vi "Pre Launch Init.vi"(11 "Cylinder in":refnum<class "Cylinder.lvclass">) -> (0 "error out":errorcluster, 3 "Cylinder out":refnum<class "Cylinder.lvclass">)   [LabVIEW 2015, in "cRIO-Carbondioxide.lvlib" / "CO2-Actor.lvlib" / "Cylinder.lvclass"]
doc: "(<B>Filename</B>: Actor Framework.lvlib:Actor.lvclass:Pre Launch Init.vi)\n\nDefines behavior that occurs after the Launch Actor method is invoked but before the actor's Actor Core method begins running.\n\nThe Pre Launch Init method is guaranteed to finish before the Launch Actor method returns to its caller and before the actor itself receives any messages. Any references that the Pre Launch Init method obtains are guaranteed to have the same lifetime as the actor itself. Any errors that the Pre Launch Init method returns will abort the launch.\n\nBy default, this method does nothing. A descendant class may override it to define behavior."
uses:
  Cylinder.lvclass
  Cylinder.lvclass/Cylinder.ctl
  <vilib>/ActorFramework/Actor/Actor.lvclass/Actor.ctl
  <vilib>/ActorFramework/Message Enqueuer/Message Enqueuer.lvclass/Message Enqueuer.ctl
  Cylinder Messages/Home Msg/Home Msg.lvclass/Home Msg.ctl
  <vilib>/ActorFramework/Actor/Read Self Enqueuer.vi
  <vilib>/ActorFramework/Message Enqueuer/Enqueue.vi
  <vilib>/ActorFramework/Message Enqueuer/Init from Existing Queue.vi
  <vilib>/ActorFramework/Message Priority Queue/Priority Enqueue.vi
  CO2 Actor/CO2 Actor.lvclass
  Cylinder Messages/Home Msg/Home Msg.lvclass
  Interlocks/Interlock Chain/Interlock Chain.lvclass
  CO2 Actor Messages/Launch Nested Actors Msg/Launch Nested Actors Msg.lvclass
  <vilib>/ActorFramework/Message Enqueuer/Message Enqueuer.lvclass
  <vilib>/ActorFramework/Actor/Actor.lvclass
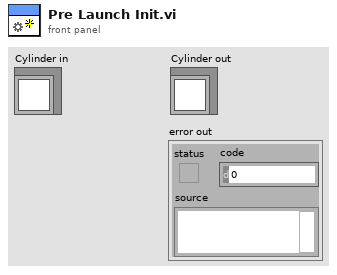
[diagram p1: front panel]
types:
  T1 = cluster{"Read Access":enum8{"Allowed", "Required", "None"}, "Write Access":enum8{"Allowed", "Required", "None"}}
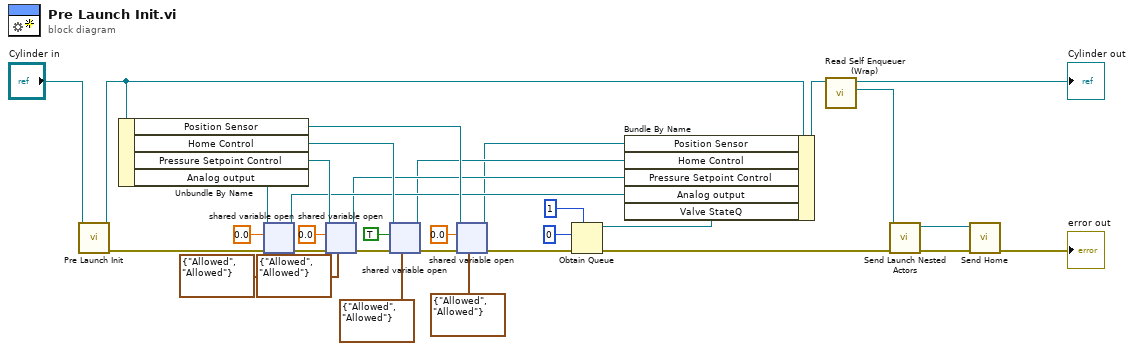
[diagram p0: block diagram]
diagram:
  n1 = call-parent "Pre Launch Init.vi"("CO2 Actor in"="Cylinder in") -> ("error out"=w30:errorcluster, "CO2 Actor out"=w26:refnum<class "Cylinder.lvclass">)  [unwired: 9 in]
  n2 = Unbundle By Name(w26) -> ("Position Sensor"=w9:refnum<k21>, "Home Control"=w16:refnum<k21>, "Pressure Setpoint Control"=w27:refnum<k21>, "Analog output"=w29:refnum<k21>)
  n3 = shared-variable-open(w29, w30, 0.0 ("data type"), T1 {"Read Access"=enum."Allowed", "Write Access"=enum."Allowed"} ("access")) -> (w5:refnum<k21>, w28:errorcluster)
  n4 = shared-variable-open(w27, w28, 0.0, T1 {"Read Access"=enum."Allowed", "Write Access"=enum."Allowed"} ("access")) -> (w4:refnum<k21>, w17:errorcluster)
  n5 = shared-variable-open(w16, w17, TRUE, T1 {"Read Access"=enum."Allowed", "Write Access"=enum."Allowed"} ("access")) -> (w3:refnum<k21>, w10:errorcluster)
  n6 = shared-variable-open(w9, w10, 0.0 ("data type"), T1 {"Read Access"=enum."Allowed", "Write Access"=enum."Allowed"} ("access")) -> (w2:refnum<k21>, w6:errorcluster)
  n7 = Obtain Queue(max queue size (-1, unlimited)=1, element data type=u16 0 ("element"), error in (no error)=w6) -> (queue out=w1:refnum<queue>, error out=w19:errorcluster)  [unwired: 2 in, 1 out]
  n8 = Bundle By Name(cluster=w26, "Position Sensor"=w2, "Home Control"=w3, "Pressure Setpoint Control"=w4, "Analog output"=w5, "Valve StateQ"=w1) -> (w21:refnum<class "Cylinder.lvclass">)
  n9 = call "Read Self Enqueuer (Wrap).vi"("CO2 Actor in"=w21) -> ("Actor Framework:Message Enqueuer"=w18:refnum<class "Message Enqueuer.lvclass">, "CO2 Actor out"=→"Cylinder out":refnum<class "Cylinder.lvclass">)  [unwired: 9 in]
  n10 = call "Send Launch Nested Actors.vi"("error in (no error)"=w19, "Message Enqueuer"=w18) -> ("error out"=w13:errorcluster, "Message Enqueuer out"=w11:refnum<class "Message Enqueuer.lvclass">)  [unwired: 8 in]
  n11 = call "Send Home.vi"("error in (no error)"=w13, "Message Enqueuer"=w11) -> ("error out"=→"error out":errorcluster)  [unwired: 8 in, 1 out]
